vi "MeasureBigIV.vi"(0 ".NET Refnum in":refnum<k24>, 1 ".NET Refnum":refnum<k24>, 2 "Junction Name":string, 5 "MaxVoltage":dbl, 7 "appended path":path, 12 "new file path (Not A Path if cancelled)":path, 13 "UiDefinition":T1, 14 "Function":string) -> (15 "error out":errorcluster)   [LabVIEW 2020]
uses:
  C:/Users/User/Desktop/Automation/CurrentVersion/LabviewDXFViewer/bin/Release/LabviewDXFViewer.exe
  LabviewDXFViewer/bin/Release/LabviewDXFViewer.exe
  UIReferences.ctl
  <vilib>/Utility/file.llb/Write Delimited Spreadsheet (DBL).vi
  <vilib>/Utility/file.llb/Write Delimited Spreadsheet (string).vi
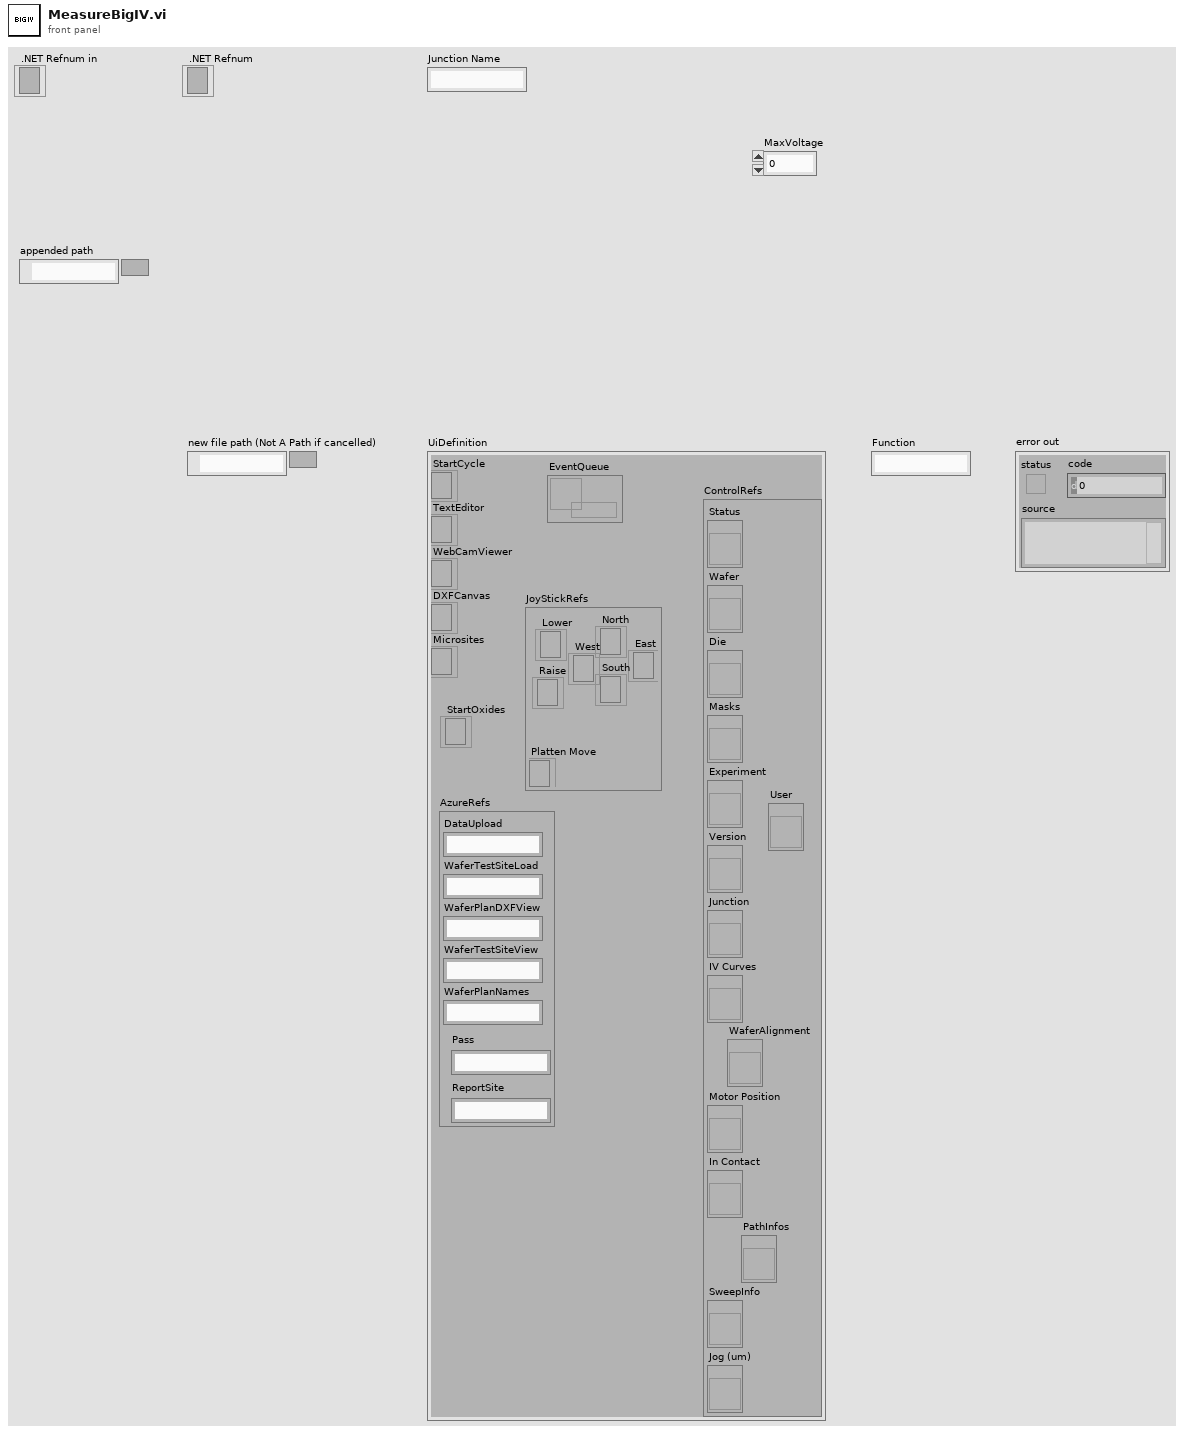
[diagram p1: front panel]
types:
  T1 = typedef "UIReferences.ctl" = cluster{"StartCycle":refnum<k24>, "TextEditor":refnum<k24>, "WebCamViewer":refnum<k24>, "DXFCanvas":refnum<k24>, "Microsites":refnum<k24>, "JoyStickRefs":cluster{"North":refnum<k24>, "Lower":refnum<k24>, "Raise":refnum<k24>, "Platten Move":refnum<k24>, "West":refnum<k24>, "East":refnum<k24>, "South":refnum<k24>}, "AzureRefs":cluster{"DataUpload":string, "WaferTestSiteLoad":string, "WaferPlanDXFView":string, "WaferTestSiteView":string, "WaferPlanNames":string, "Pass":string, "ReportSite":string}, "ControlRefs":cluster{"Status":refnum<vi>, "Wafer":refnum<vi>, "Die":refnum<vi>, "Masks":refnum<vi>, "Experiment":refnum<vi>, "Version":refnum<vi>, "Junction":refnum<vi>, "IV Curves":refnum<vi>, "Motor Position":refnum<vi>, "In Contact":refnum<vi>, "SweepInfo":refnum<vi>, "Jog (um)":refnum<vi>, "PathInfos":refnum<vi>, "User":refnum<vi>, "WaferAlignment":refnum<vi>}, "EventQueue":refnum<queue>, "StartOxides":refnum<k24>}
  T2 = cluster{"Current Range":dbl, "Source Measure Unit Channel (0: Channel A)":i32, "Waveform":waveform(dbl), "VISA resource name":refnum<visa-resource-name>, "CodeText":string}
  T3 = typedef "CapacitanceInfos.ctl" = cluster{"Conductance":dbl, "CapacitanceIV":dbl, "Intercept":dbl, "CapacitanceSW":dbl, "Sum":dbl, "CapacitanceInfos":T4[], "CapacitancePhase":dbl, "dC/dV":dbl, "Function":string, "OtherInfo":dbl[][]}
  T4 = typedef "CapacitanceRecord.ctl" = cluster{"Freq":dbl, "Vpp":dbl, "PhaseS":dbl, "Irms":dbl, "PhaseC":dbl, "Theta":dbl, "VDrive":dbl, "Capacitance":dbl, "Other":dbl}
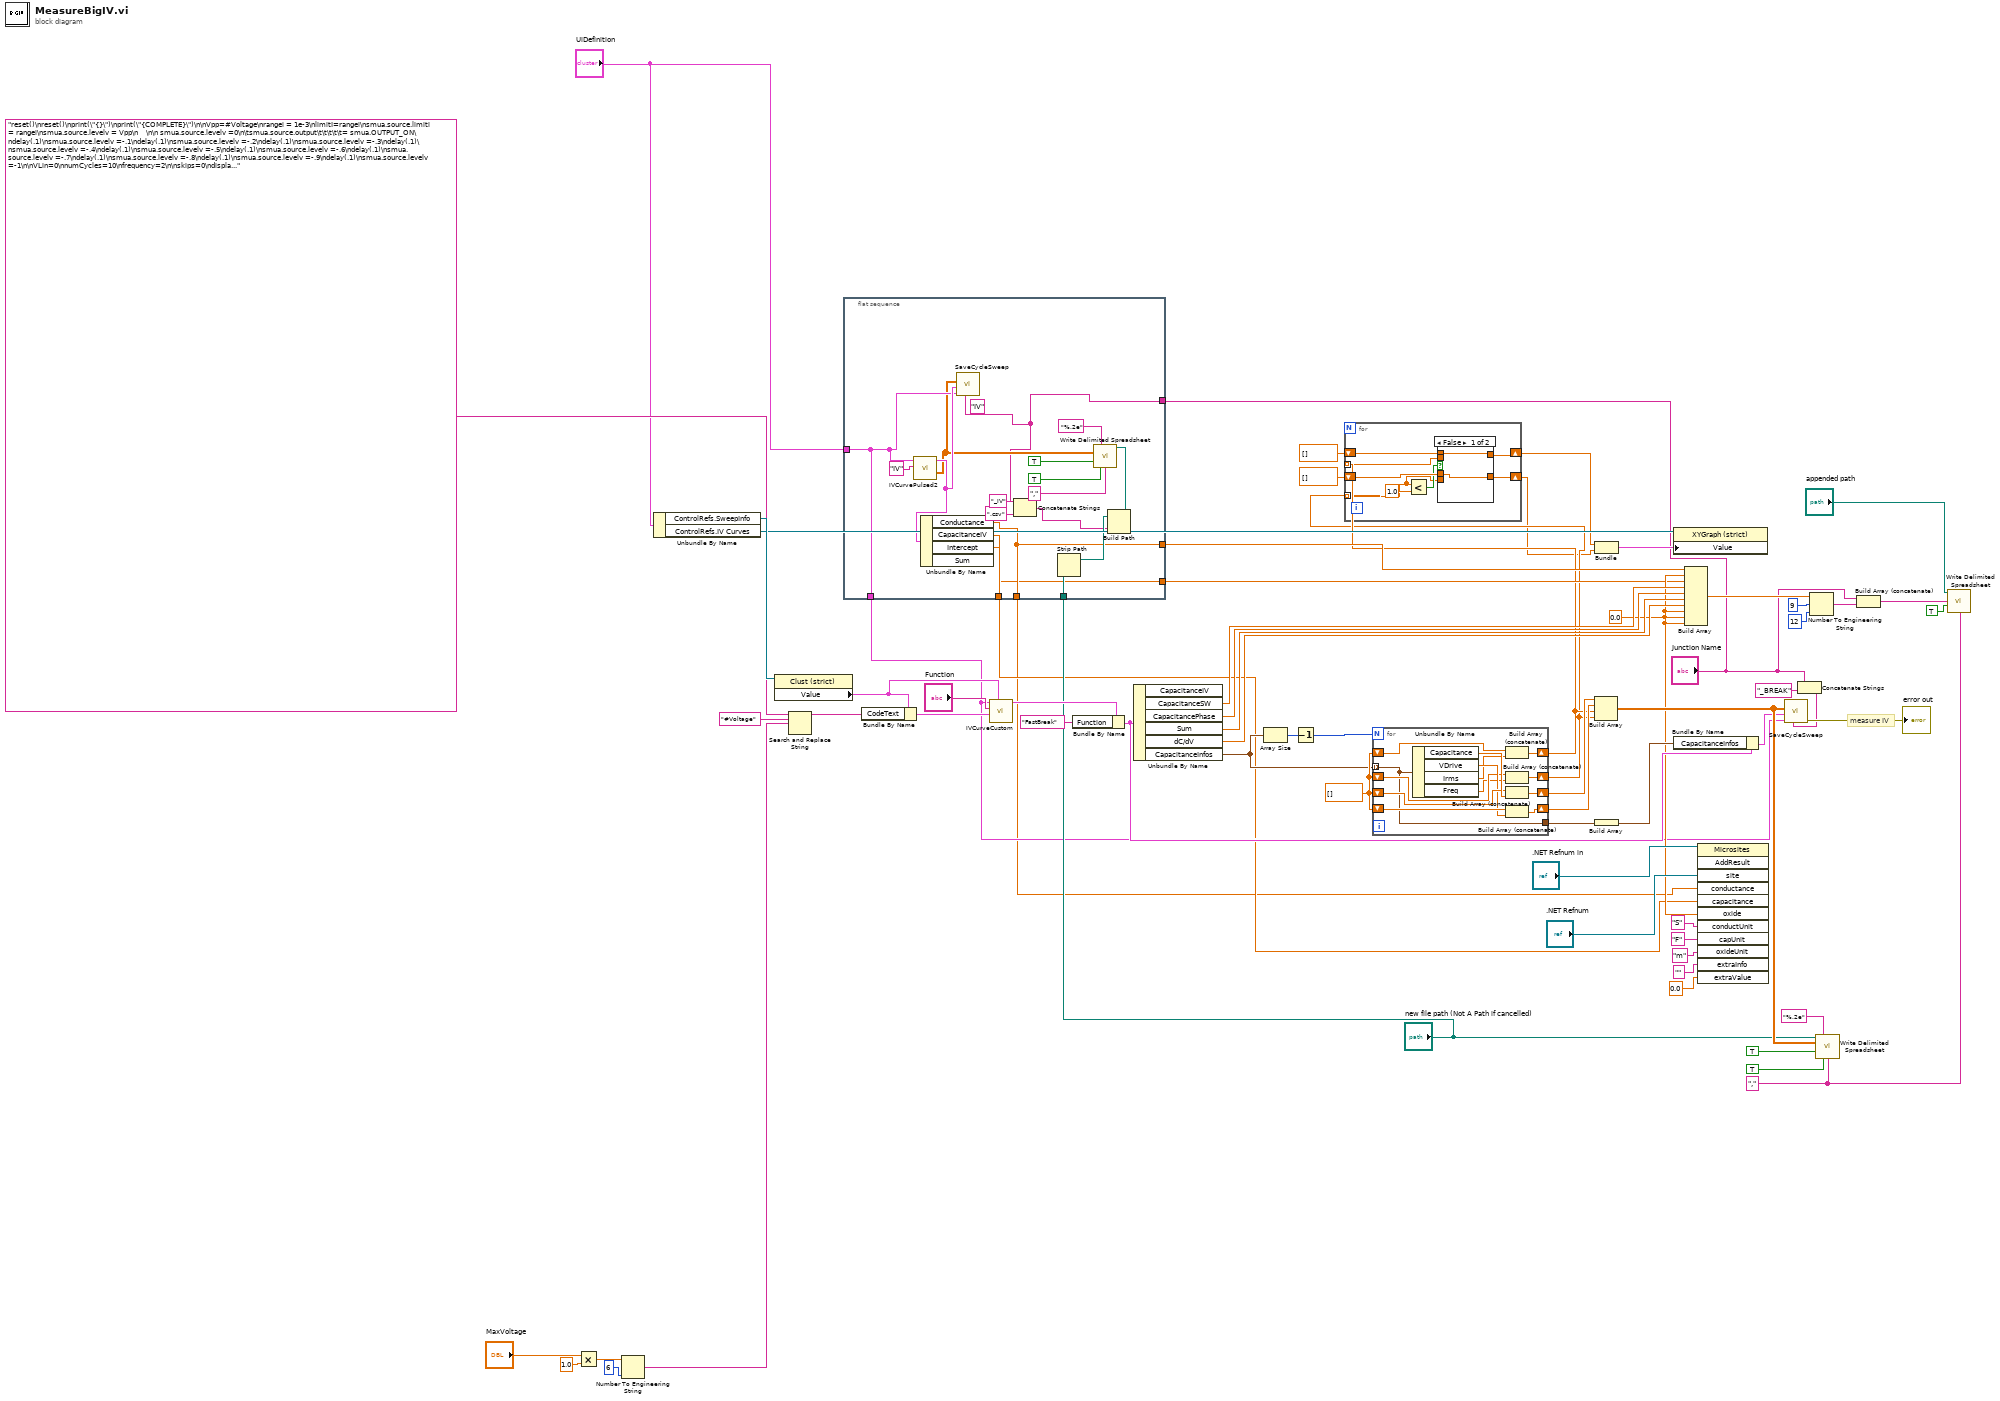
[diagram p0: block diagram]
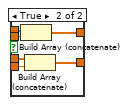
[diagram p2: hidden frame]
diagram:
  w40 = dbl[] []
  w20 = 0.0 ("element")
  w47 = "," ("delimiter (\\t)")
  # "measure IV"
  n1 = Multiply(x="MaxVoltage", y=1.0) -> (x*y=w27:dbl)
  n2 = Number To Engineering String(2:i16 6 ("precision (6)"), 4:w27) -> (0:w25:string)  [unwired: 2 in]
  n3 = Unbundle By Name("UiDefinition") -> ("ControlRefs.SweepInfo"=w45:refnum<vi>, "ControlRefs.IV Curves"=w41:refnum<vi>)
  n4 = property class="Clust (strict)"(reference=w45) -> ("Value"=w28:T2)  [unwired: 1 in, 2 out]
  n5 = Search and Replace String(input string="reset()\nreset()\nprint(\"{}\")\nprint(\"{COMPLETE}\")\n\nVpp=#Voltage\nrangei = 1e-3\nlimitI=rangei\nsmua.source.limiti = rangei\nsmua.source.levelv = Vpp\n    \n\n smua.source.levelv =0\n\tsmua.source.output\t\t\t\t\t= smua.OUTPUT_ON\ndelay(.1)\nsmua.source.levelv =-.1\ndelay(.1)\nsmua.source.levelv =-.2\ndelay(.1)\nsmua.source.levelv =-.3\ndelay(.1)\nsmua.source.levelv =-.4\ndelay(.1)\nsmua.source.levelv =-.5\ndelay(.1)\nsmua.source.levelv =-.6\ndelay(.1)\nsmua.source.levelv =-.7\ndelay(.1)\nsmua.source.levelv =-.8\ndelay(.1)\nsmua.source.levelv =-.9\ndelay(.1)\nsmua.source.levelv =-1\n\nVLin=0\nnumCycles=10\nfrequency=2\n\nskips=0\ndisplay=1\n\n\n\tlocal COMPLETE = \"{COMPLETE}\"\n\t-- Generate the source values\n\n\tlocal sourceValues\t\t= {} \n\tlocal pointsPerCycle\t= 60 / frequency\n\tlocal pointsPer60 = 1\n\tlocal numDataPoints\t\t= pointsPerCycle * numCycles\n\n\n\tp=(Vpp+1)/numDataPoints\n    for i = 1, numDataPoints do\n        sourceValues[i] =(i-1)*p-1\n      \n    end\n\n\t-- Configure the SMU ranges\n\tsmua.reset()\n\tsmua.source.settling\t\t= smua.SETTLE_FAST_POLARITY\n\tsmua.source.autorangev\t\t= smua.AUTORANGE_OFF\n\tsmua.source.autorangei\t\t= smua.AUTORANGE_OFF\nsmua.source.rangev\t\t\t= 10\n smua.source.limitv\t\t= 10\n\tsmua.source.delay\t\t\t= 0\n\tsmua.source.limiti\t\t\t=1e-3\n\n\tsmua.measure.autorangev\t\t= smua.AUTORANGE_OFF\n\tsmua.measure.autorangei\t\t= smua.AUTORANGE_OFF\n\tsmua.measure.autozero\t\t= smua.AUTOZERO_OFF\n\tsmua.measure.delay\t\t\t= 0\n\tsmua.measure.delayfactor    = 1\n\tsmua.measure.analogfilter   = 0\n\n\t-- Voltage will be measured on the same range as the source range\n\tsmua.measure.rangei\t\t\t=limitI\n\tsmua.measure.nplc\t\t\t=1\n\n\t-- Prepare the Reading Buffers\n\tsmua.nvbuffer1.clear()\n\tsmua.nvbuffer1.collecttimestamps\t= 1\n\tsmua.nvbuffer2.clear()\n\tsmua.nvbuffer2.collecttimestamps\t= 1\n\n\t-- Configure the trigger model\n\t--============================\n\t\n\t-- Timer 1 controls the time between source points\n\ttrigger.timer[1].delay = (1 / 60)\n\ttrigger.timer[1].passthrough = true\n\ttrigger.timer[1].stimulus = smua.trigger.ARMED_EVENT_ID\n\ttrigger.timer[1].count = numDataPoints - 1\n\n\t-- Configure the SMU trigger model\n\tsmua.trigger.source.listv(sourceValues)\n\tsmua.trigger.source.limiti\t\t= limitI\n\tsmua.trigger.measure.action\t\t= smua.ENABLE\n\tsmua.trigger.measure.iv(smua.nvbuffer1, smua.nvbuffer2)\n\tsmua.trigger.endpulse.action\t= smua.SOURCE_HOLD\n\tsmua.trigger.endsweep.action\t= smua.SOURCE_IDLE\n\tsmua.trigger.count\t\t\t\t= numDataPoints\n\tsmua.trigger.arm.stimulus\t\t= 0\n\tsmua.trigger.source.stimulus\t= trigger.timer[1].EVENT_ID\n\tsmua.trigger.measure.stimulus\t= 0\n\tsmua.trigger.endpulse.stimulus\t= 0\n\tsmua.trigger.source.action\t\t= smua.ENABLE\n\t-- Ready to begin the test\n\n\tsmua.source.output\t\t\t\t\t= smua.OUTPUT_ON\n\t-- Start the trigger model execution\n\tsmua.trigger.initiate()\n\t-- Wait until the sweep has completed\n\twaitcomplete()\n\tsmua.source.output\t\t\t\t\t= smua.OUTPUT_OFF\n\n\t-- Print the data back to the Console in tabular format\n\nfor x=1, smua.nvbuffer2.n,pointsPer60 do\n     if (smua.nvbuffer2[x]>.008) then\n         print(smua.nvbuffer1[x], 1, 1.0/60,smua.nvbuffer1.timestamps[x] ,0 , 0, sourceValues[x],smua.nvbuffer2[x],0)\n     end\n\tend\n\nprint(\"{COMPLETE}\")\n\nsmua.source.output = smua.OUTPUT_OFF" ("CodeText"), search string="#Voltage", replace string=w25) -> (result string=w32:string)  [unwired: 5 in, 3 out]
  n6 = flat-sequence {
    tunnel: "new file path (Not A Path if cancelled)" -> [w80]
    tunnel: "UiDefinition" -> [w73]
    tunnel: [w73] -> w14
    tunnel: [w77] -> w13
    tunnel: [w76] -> w12
    tunnel: [w76] -> w11
    tunnel: [w75] -> w10
    tunnel: "Junction Name" -> [w68]
    frame #0 {
      (unwired) "IV" ("string")
      n7 = call "IVCurvePulsed2.vi"("Program"="IV", "UiDefinition"=w73) -> ("appended array"=w72:dbl[][], "InfoCluster"=w74:T3)  [unwired: 8 in]
      n8 = Unbundle By Name(w74) -> ("Conductance"=w76:dbl, "CapacitanceIV"=w77:dbl, "Intercept"=w75:dbl)  [unwired: 1 out]
      n9 = call "SaveCycleSweep.vi"("JunctionName"=w68, "UiDefinition 2"=w73, "InfoCluster"=w74, "appended array"=w72) -> ()  [unwired: 7 in, 1 out]
      n10 = Concatenate Strings(w68, "_IV" ("string"), ".csv" ("string")) -> (w70:string)
      n11 = Strip Path(path=w80) -> (stripped path=w78:path)  [unwired: 1 out]
      n12 = Build Path(base path=w78, name or relative path=w70) -> (appended path=w79:path)
      n13 = call-poly <vilib>:"Write Delimited Spreadsheet.vi"("file path (dialog if empty)"=w79, "format (%.3f)"="%.2e", "2D data"=w72, "append to file? (new file:F)"=TRUE, "transpose? (no:F)"=TRUE, "delimiter (\\t)"="," ("delimiter (\\t)")) -> ()  [unwired: 8 in, 2 out]
    }
  }
  n14 = Bundle By Name(cluster=w28, "CodeText"=w32) -> (w31:T2)
  n15 = call "IVCurveCustom.vi"("OriginalSweepInfo"=w28, "SweepInfo"=w31, "Program"="Function", "UiDefinition"=w14) -> ("InfoCluster"=w29:T3)  [unwired: 6 in, 1 out]
  n16 = Bundle By Name(cluster=w29, "Function"="FastBreak") -> (w44:T3)
  n17 = Unbundle By Name(w44) -> ("CapacitanceSW"=w60:dbl, "CapacitancePhase"=w61:dbl, "Sum"=w58:dbl, "dC/dV"=w59:dbl, "CapacitanceInfos"=w19:T4[])  [unwired: 1 out]
  n18 = Array Size(array=w19) -> (size(s)=w18:i32)
  n19 = Decrement(x=w18) -> (x-1=w17:i32)
  n20 = for {
    N: w17 -> [_]
    tunnel: w19 -> [w86] mode=indexing
    shift-right: [w98] -> w37
    shift-left: w40 -> [w96]
    shift-right: [w95] -> w39
    shift-left: w40 -> [w94]
    shift-right: [w91] -> w8
    shift-left: w40 -> [w92]
    shift-right: [w89] -> w7
    shift-left: w40 -> [w90]
    tunnel: [w86] -> w22
    n21 = Unbundle By Name(w86) -> ("Capacitance"=w97:dbl, "VDrive"=w93:dbl, "Irms"=w88:dbl, "Freq"=w87:dbl)
    n22 = Build Array (concatenate)(w92, w88) -> (w91:dbl[])
    n23 = Build Array (concatenate)(w90, w87) -> (w89:dbl[])
    n24 = Build Array (concatenate)(w96, w97) -> (w98:dbl[])
    n25 = Build Array (concatenate)(w94, w93) -> (w95:dbl[])
  }
  n26 = for {
    tunnel: w8 -> [w99] mode=indexing
    tunnel: w7 -> [w100] mode=indexing
    shift-right: [w106] -> w3
    shift-left: dbl[] [] -> [w104]
    shift-right: [w105] -> w4
    shift-left: dbl[] [] -> [w103]
    n27 = Less?(x=w100, y=1.0) -> (x < y?=w101:bool)
    n28 = case shown="False" w101 {
      tunnel: [w107 w114] -> w106
      tunnel: [w108 w113] -> w105
      tunnel: w104 -> [w107 w112]
      tunnel: w103 -> [w108 w111]
      tunnel: w100 -> [_ w110]
      tunnel: w99 -> [_ w109]
      frame False {
      }
      frame True {
        n29 = Build Array (concatenate)(w111, w109) -> (w113:dbl[])
        n30 = Build Array (concatenate)(w112, w110) -> (w114:dbl[])
      }
    }
  }
  n31 = Build Array(w37, w39, w8, w7) -> (w38:dbl[][])
  n32 = Bundle(w4, w3) -> (w36:cluster{dbl[], dbl[]})  [unwired: 1 in]
  n33 = Build Array(w22) -> (w21:T4[])
  n34 = property class="XYGraph (strict)"(reference=w41, "Value"=w36) -> ()  [unwired: 1 in, 2 out]
  n35 = Bundle By Name(cluster=w44, "CapacitanceInfos"=w21) -> (w23:T3)
  n36 = Build Array(w11, w20, w10, w60, w61, w58, w59, w20, w20, w20) -> (w57:dbl[])
  n37 = invoke class="Microsites" method="AddResult"(reference=".NET Refnum in", "site"=".NET Refnum", "conductance"=w12, "capacitance"=w13, "oxide"=w20, "conductUnit"="S", "capUnit"="F", "oxideUnit"="m" ("interceptUnit"), "extraInfo"="", "extraValue"=0.0) -> ()  [unwired: 2 in, 12 out]
  n38 = Concatenate Strings("Junction Name", "_BREAK" ("string")) -> (w2:string)
  n39 = call "SaveCycleSweep.vi"("JunctionName"=w2, "UiDefinition 2"=w14, "InfoCluster"=w23, "appended array"=w38) -> ("error out"=→"error out":errorcluster)  [unwired: 7 in]
  n40 = Number To Engineering String(2:i16 12 ("precision (6)"), 3:i16 9 ("width (-)"), 4:w57) -> (0:w50:string[])  [unwired: 1 in]
  n41 = call-poly <vilib>:"Write Delimited Spreadsheet.vi"("file path (dialog if empty)"="new file path (Not A Path if cancelled)", "format (%.3f)"="%.2e", "2D data"=w38, "append to file? (new file:F)"=TRUE, "transpose? (no:F)"=TRUE, "delimiter (\\t)"=w47) -> ()  [unwired: 8 in, 2 out]
  n42 = Build Array (concatenate)("Junction Name", w50) -> (w52:string[])
  n43 = call-poly <vilib>:"Write Delimited Spreadsheet.vi"("file path (dialog if empty)"="appended path", "1D data"=w52, "append to file? (new file:F)"=TRUE, "delimiter (\\t)"=w47) -> ()  [unwired: 10 in, 2 out]
